vi "ShowScrollBar.vi"(8 "Origin in":T1, 9 "Task":enum16{"Read", "Change", "Reset"}(ring)=enum."Reset", 11 "VI in":refnum<vi>) -> (0 "Origin":T1)   [LabVIEW 2016]
uses:
  <vilib>/Utility/miscctls.llb/LVPointTypeDef.ctl
  <vilib>/Utility/miscctls.llb/LVRectTypeDef.ctl
panel:
  out "InitialBounds":T2
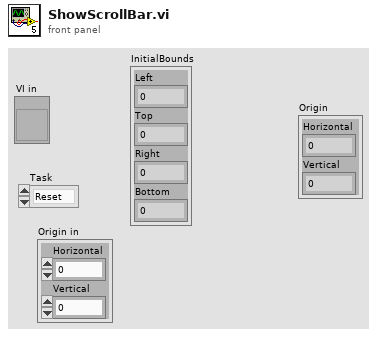
[diagram p1: front panel]
types:
  T1 = typedef "LVPointTypeDef.ctl" = cluster{"Horizontal":i16, "Vertical":i16}
  T2 = typedef "LVRectTypeDef.ctl" = cluster{"Left":i16, "Top":i16, "Right":i16, "Bottom":i16}
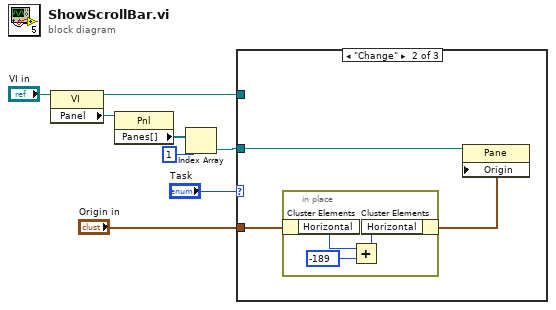
[diagram p0: block diagram]
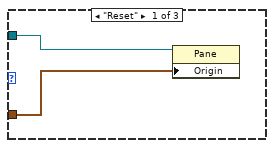
[diagram p2: hidden frame]
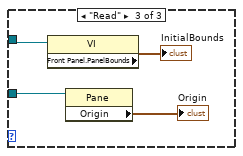
[diagram p3: hidden frame]
diagram:
  n1 = property class="VI"(reference="VI in") -> (reference out=w4:refnum<vi>, "Panel"=w6:refnum<vi>)  [unwired: 1 in, 1 out]
  n2 = property class="Pnl"(reference=w6) -> ("Panes[]"=w7:refnum<vi>[])  [unwired: 1 in, 2 out]
  n3 = Index Array(array=w7, index=1) -> (element=w5:refnum<vi>)
  n4 = case shown="\"Change\"" "Task" {
    tunnel: w5 -> [w10 w13 w20]
    tunnel: w4 -> [_ _ w19]
    tunnel: "Origin in" -> [w9 w12 _]
    frame "Reset" {
      n5 = property class="Pane"(reference=w10, "Origin"=w9) -> ()  [unwired: 1 in, 2 out]
    }
    frame "Change" {
      n6 = in-place {
        n7 = in-place-cluster #1(w12) -> ("Horizontal"=w16:i16)
        n8 = Add(x=w16, y=i16 -189) -> (x+y=w14:i16)
        n9 = in-place-cluster #1("Horizontal"=w14) -> (w11:T1)
      }
      n10 = property class="Pane"(reference=w13, "Origin"=w11) -> ()  [unwired: 1 in, 2 out]
    }
    frame "Read" {
      n11 = property class="VI"(reference=w19) -> ("Front Panel.PanelBounds"=→"InitialBounds":T2)  [unwired: 1 in, 2 out]
      n12 = property class="Pane"(reference=w20) -> ("Origin"=→"Origin":T1)  [unwired: 1 in, 2 out]
    }
  }
